vi "Create-client-application.vi"(8 "error in (no error)":errorcluster, 9 "Module path":path=path "C:/Users/Christoph/Desktop/2015-05-23 - SLM - STORM/builds/SLMTools/PowderDeposition.lvlibp", 10 "Module type":T1=enum."PowderDeposition", 11 "ModComm in":T2) -> (0 "error out":errorcluster, 3 "ModComm out":T2)   [LabVIEW 2013, in "SLMServer.lvlib" / "SLMServer.lvclass"]
uses:
  SLMServer.lvclass
  Object-reference.ctl
  Supported-module-types.ctl
  UI-messages.ctl
  SLMServer.lvclass/SLMServer.ctl
  Read Server channel.vi
  SA-SLMAPI/Sources/Message.lvclass
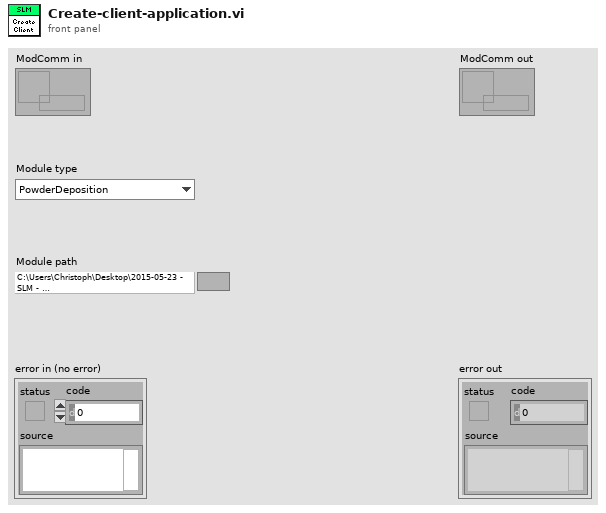
[diagram p1: front panel]
types:
  T1 = typedef "SLMServer.lvlib/SLMServer.lvclass/Supported-module-types.ctl" = enum16{"SLMControl", "PowderDeposition", "CameraVision", "Server", "All", "StrategyParser", "MaterialCharacterization", "StatusMonitor", "SLMSimulation", "LaserCharacterization"}
  T2 = typedef "SLMServer.lvlib/SLMServer.lvclass/Object-reference.ctl" = refnum<data-value>
  T3 = typedef "SLMServer.lvlib/SLMServer.lvclass/UI-messages.ctl" = enum16{"Time out", "User cancel", "Module cancel", "Client inactivity", "Client limit", "Client started"}
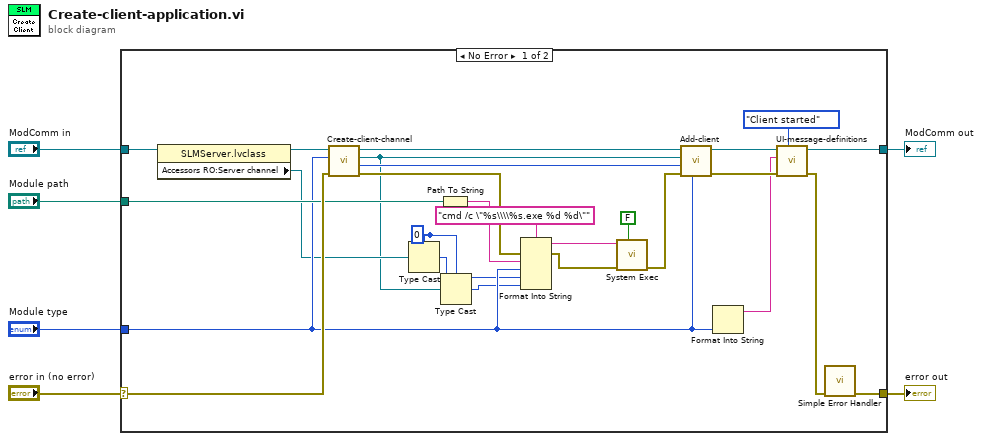
[diagram p0: block diagram]
diagram:
  n1 = case shown="No Error" "error in (no error)" {
    selector: "error in (no error)" -> [w21 w34]
    tunnel: [w23 w34] -> w5
    tunnel: [w24 w33] -> w3
    tunnel: "ModComm in" -> [w22 w33]
    tunnel: "Module path" -> [w14 _]
    tunnel: "Module type" -> [w13 _]
    frame No Error {
      w9 = 0
      n2 = property class="SLMServer.lvclass"(reference=w22) -> (reference out=w32:T2, "Accessors RO:Server channel"=w11:refnum<queue>)  [unwired: 1 in, 1 out]
      n3 = call "Create-client-channel.vi"("error in (no error)"=w21, "Client type"=w13, "ModComm in"=w32) -> ("error out"=w17:errorcluster, "Client ID"=w30:i32, "Client channel"=w7:refnum<queue>, "ModComm out"=w31:T2)  [unwired: 5 in]
      n4 = Type Cast(type=w9, x=w11) -> (*(type *) &x=w10:i32)
      n5 = Path To String(path=w14) -> (string=w12:string)
      n6 = Type Cast(type=w9, x=w7) -> (*(type *) &x=w8:i32)
      n7 = Format Into String(format string="cmd /c \"%s\\\\%s.exe %d %d\"", error in=w17, w12, w13, w10, w8) -> (resulting string=w19:string, error out=w18:errorcluster)  [unwired: 1 in]
      n8 = call <vilib>:"System Exec.vi"("wait until completion? (T)"=FALSE, "error in (no error)"=w18, "command line"=w19) -> ("error out"=w16:errorcluster)  [unwired: 5 in, 3 out]
      n9 = call "Add-client.vi"("Client type"=w13, "error in (no error)"=w16, "Client ID"=w30, "Client channel"=w7, "ModComm in"=w31) -> ("error out"=w29:errorcluster, "ModComm out"=w25:T2)  [unwired: 5 in]
      n10 = Format Into String(w13) -> (resulting string=w27:string)  [unwired: 3 in, 1 out]
      n11 = call "UI-message-definitions.vi"("Message"=UI-messages."Client started", "error in (no error)"=w29, "Additional text"=w27, "ModComm in"=w25) -> ("error out"=w28:errorcluster, "ModComm out"=w24:T2)  [unwired: 6 in]
      n12 = call <vilib>:"Simple Error Handler.vi"("error in (no error)"=w28) -> ("error out"=w23:errorcluster)  [unwired: 4 in, 4 out]
    }
    frame Error {
    }
  }
  "error out" <- w5
  "ModComm out" <- w3
